vi "Configure Trigger Model SMU Source Action.vi"(0 "VISA resource name":refnum<visa-resource-name>, 1 "Source Measure Unit Channel (0: Channel A)":i32(ring) items=["Channel A", "Channel B"], 2 "Enable Source Sweep (F: Disable)":bool, 3 "Sweep Type (0: Linear Current)":i32(ring) items=["Linear Current", "Linear Voltage", "List Current", "List Voltage", "Logarithmic Current", "Logarithmic Voltage"], 4 "Sweep Points (10)":i32=10, 5 "error in (no error)":errorcluster, 6 "Pulse Stop Level (1)":dbl=1.0, 7 "Enable Current Limit (T: Enable)":bool=TRUE, 8 "Pulse Start Level (0.1)":dbl=0.1, 9 "Source Limit (1)":dbl=1.0, 10 "Sweep List":dbl[](array[numeric]), 11 "Asymptote (0)":dbl) -> (14 "VISA resource name out":refnum<visa-resource-name>, 19 "error out":errorcluster)   [LabVIEW 2017, in "Keithley 2600 Series.lvlib"]
doc: "Configures the source action of the trigger model SMU (Source Measure Unit)."
uses:
  <instrlib>/Keithley 2600 Series/Keithley 2600 Series.lvlib
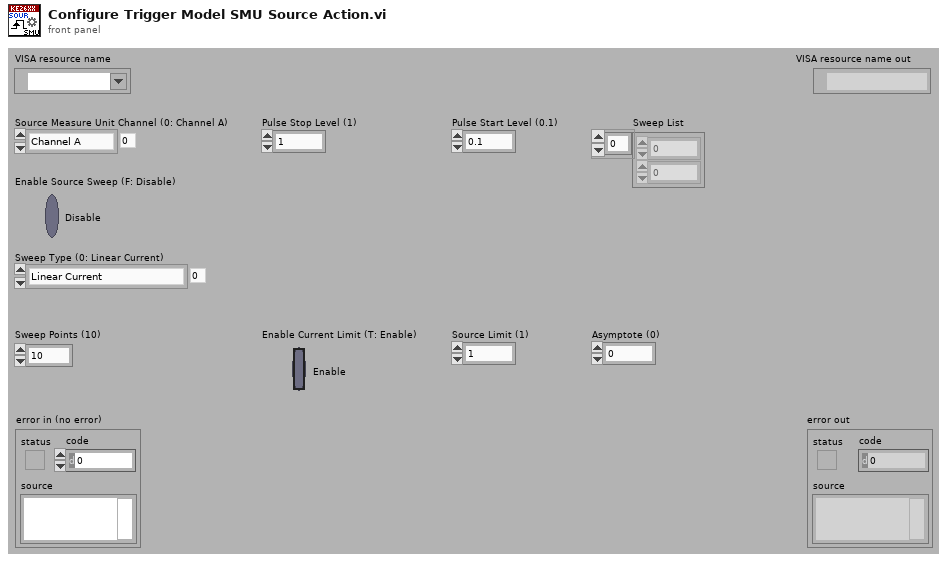
[diagram p1: front panel]
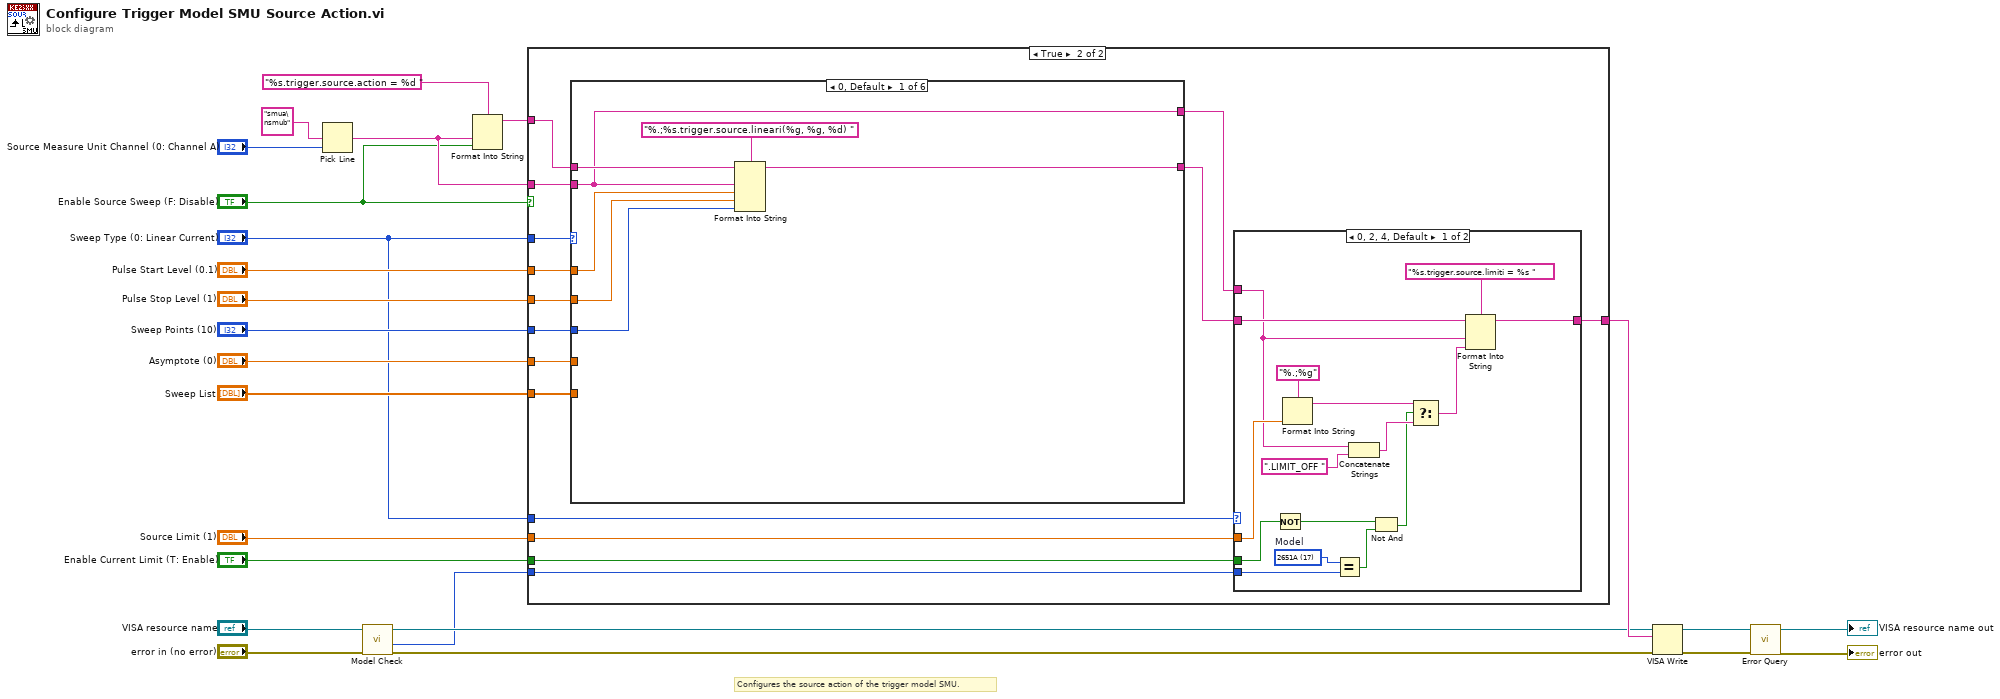
[diagram p0: block diagram]
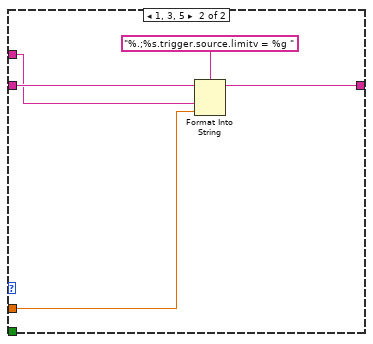
[diagram p3: hidden frame]
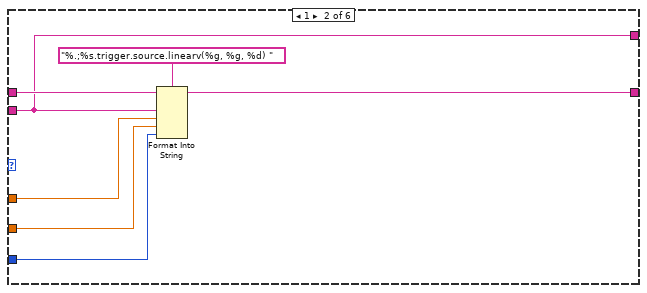
[diagram p4: hidden frame]
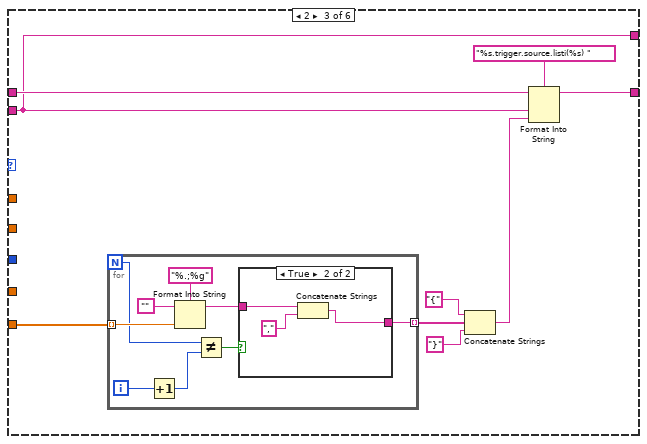
[diagram p5: hidden frame]
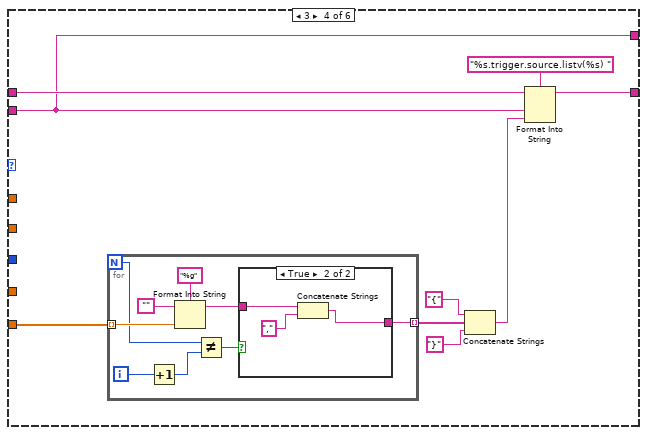
[diagram p7: hidden frame]
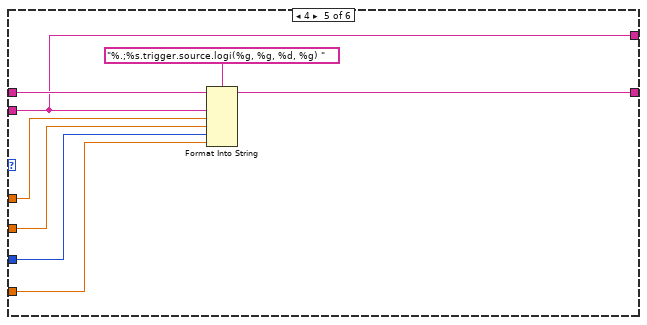
[diagram p9: hidden frame]
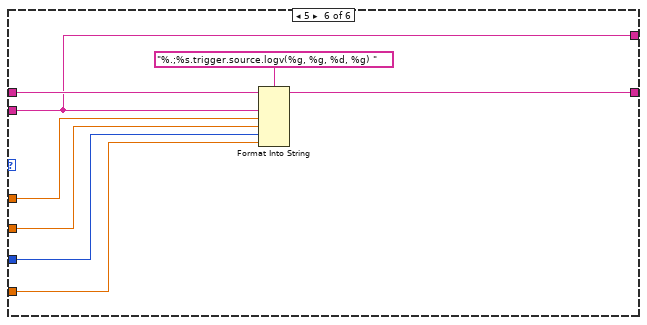
[diagram p10: hidden frame]
diagram:
  # "Configures the source action of the trigger model SMU."
  n1 = Pick Line(multi-line string="smua\nsmub", line index="Source Measure Unit Channel (0: Channel A)") -> (output string=w17:string)  [unwired: 1 in]
  n2 = call <instrlib>:"Model Check.vi"("error in (no error)"="error in (no error)", "VISA resource name"="VISA resource name") -> ("error out"=w3:errorcluster, "Model"=w2:u16, "VISA resource name out"=w4:refnum<visa-resource-name>)  [unwired: 6 in, 1 out]
  n3 = Format Into String(format string="%s.trigger.source.action = %d ", w17, "Enable Source Sweep (F: Disable)") -> (resulting string=w12:string)  [unwired: 2 in, 1 out]
  n4 = case shown="True" "Enable Source Sweep (F: Disable)" {
    tunnel: w17 -> [_ w28]
    tunnel: [w25 w29] -> w7
    tunnel: "Sweep Type (0: Linear Current)" -> [_ w40]
    tunnel: "Pulse Start Level (0.1)" -> [_ w39]
    tunnel: "Pulse Stop Level (1)" -> [_ w38]
    tunnel: "Sweep Points (10)" -> [_ w37]
    tunnel: "Sweep List" -> [_ w36]
    tunnel: w12 -> [w25 w35]
    tunnel: "Asymptote (0)" -> [_ w34]
    tunnel: "Sweep Type (0: Linear Current)" -> [_ w32]
    tunnel: "Enable Current Limit (T: Enable)" -> [_ w31]
    tunnel: "Source Limit (1)" -> [_ w30]
    tunnel: w2 -> [_ w26]
    frame False {
    }
    frame True {
      n5 = case shown="0, Default" w40 {
        tunnel: w28 -> [w62 w69 w76 w103 w120 w128]
        tunnel: w39 -> [w67 w74 _ _ w125 w131]
        tunnel: w38 -> [w66 w73 _ _ w124 w132]
        tunnel: w37 -> [w65 w72 _ _ w123 w133]
        tunnel: w36 -> [_ _ w80 w99 _ _]
        tunnel: w35 -> [w64 w71 w78 w105 w127 w130]
        tunnel: w34 -> [_ _ _ _ w122 w134]
        tunnel: [w63 w70 w77 w104 w121 w129] -> w33
        tunnel: [w62 w69 w76 w103 w120 w128] -> w27
        frame 0, Default {
          n6 = Format Into String(format string="%.;%s.trigger.source.lineari(%g, %g, %d) ", initial string=w64, w62, w67, w66, w65) -> (resulting string=w63:string)  [unwired: 1 in, 1 out]
        }
        frame 1 {
          n7 = Format Into String(format string="%.;%s.trigger.source.linearv(%g, %g, %d) ", initial string=w71, w69, w74, w73, w72) -> (resulting string=w70:string)  [unwired: 1 in, 1 out]
        }
        frame 2 {
          n8 = for {
            N -> [w85]
            tunnel: w80 -> [w93] mode=indexing
            tunnel: [w86] -> w83 mode=indexing
            i -> [w90]
            n9 = Increment(x=w90) -> (x+1=w89:i32)
            n10 = Format Into String(format string="%.;%g", initial string="" ("Empty String Constant"), w93) -> (resulting string=w87:string)  [unwired: 1 in, 1 out]
            n11 = Not Equal?(x=w85, y=w89) -> (x != y?=w88:bool)
            n12 = case shown="True" w88 {
              tunnel: w87 -> [w94 w97]
              tunnel: [w94 w95] -> w86
              frame False {
              }
              frame True {
                n13 = Concatenate Strings(w97, ",") -> (w95:string)
              }
            }
          }
          n14 = Concatenate Strings("{" ("string"), w83, "}") -> (w79:string)
          n15 = Format Into String(format string="%s.trigger.source.listi(%s) ", initial string=w78, w76, w79) -> (resulting string=w77:string)  [unwired: 1 in, 1 out]
        }
        frame 3 {
          n16 = for {
            N -> [w107]
            tunnel: w99 -> [w115] mode=indexing
            tunnel: [w108] -> w102 mode=indexing
            i -> [w112]
            n17 = Increment(x=w112) -> (x+1=w111:i32)
            n18 = Format Into String(format string="%g", initial string="" ("Empty String Constant"), w115) -> (resulting string=w109:string)  [unwired: 1 in, 1 out]
            n19 = Not Equal?(x=w107, y=w111) -> (x != y?=w110:bool)
            n20 = case shown="True" w110 {
              tunnel: w109 -> [w116 w119]
              tunnel: [w116 w117] -> w108
              frame False {
              }
              frame True {
                n21 = Concatenate Strings(w119, ",") -> (w117:string)
              }
            }
          }
          n22 = Concatenate Strings("{" ("string"), w102, "}") -> (w98:string)
          n23 = Format Into String(format string="%s.trigger.source.listv(%s) ", initial string=w105, w103, w98) -> (resulting string=w104:string)  [unwired: 1 in, 1 out]
        }
        frame 4 {
          n24 = Format Into String(format string="%.;%s.trigger.source.logi(%g, %g, %d, %g) ", initial string=w127, w120, w125, w124, w123, w122) -> (resulting string=w121:string)  [unwired: 1 in, 1 out]
        }
        frame 5 {
          n25 = Format Into String(format string="%.;%s.trigger.source.logv(%g, %g, %d, %g) ", initial string=w130, w128, w131, w132, w133, w134) -> (resulting string=w129:string)  [unwired: 1 in, 1 out]
        }
      }
      n26 = case shown="0, 2, 4, Default" w32 {
        tunnel: w33 -> [w49 w60]
        tunnel: w31 -> [w44 _]
        tunnel: w27 -> [w47 w59]
        tunnel: w30 -> [w53 w58]
        tunnel: [w55 w57] -> w29
        tunnel: w26 -> [w46 _]
        frame 0, 2, 4, Default {
          w41 = u16 17 items=["2601A", "2602A", "2611A", "2612A", "2635A", "2636A", "2657A", "2601B", "2602B", "2604B", "2606B", "2611B", "2612B", "2614B", "2634B", "2635B", "2636B", "2651A"]  # Model
          n27 = Not(x=w44) -> (.not. x?=w43:bool)
          n28 = Format Into String(format string="%.;%g", w53) -> (resulting string=w52:string)  [unwired: 2 in, 1 out]
          n29 = Equal?(x=w41, y=w46) -> (x = y?=w45:bool)
          n30 = Concatenate Strings(w47, ".LIMIT_OFF ") -> (w48:string)
          n31 = Not And(1:w45, 2:w43) -> (0:w42:bool)
          n32 = Select(t=w52, s=w42, f=w48) -> (s? t:f=w54:string)
          n33 = Format Into String(format string="%s.trigger.source.limiti = %s ", initial string=w49, w47, w54) -> (resulting string=w55:string)  [unwired: 1 in, 1 out]
        }
        frame 1, 3, 5 {
          n34 = Format Into String(format string="%.;%s.trigger.source.limitv = %g ", initial string=w60, w59, w58) -> (resulting string=w57:string)  [unwired: 1 in, 1 out]
        }
      }
    }
  }
  n35 = VISA Write(VISA resource name=w4, write buffer=w7, error in (no error)=w3) -> (VISA resource name out=w24:refnum<visa-resource-name>, error out=w23:errorcluster)  [unwired: 1 out]
  n36 = call <instrlib>:"Error Query.vi"("error in (no error)"=w23, "VISA resource name"=w24) -> ("error out"=→"error out":errorcluster, "VISA resource name out"=→"VISA resource name out":refnum<visa-resource-name>)  [unwired: 6 in, 2 out]
